vi "Simple TCP - Client_draft 1.vi"() -> ()   [LabVIEW 2021]
doc: "Demonstrates how to open a connection to an TCP server, read the data being sent, and display the data on a chart. This VI is designed to stop if the TCP connection is terminated."
uses:
  <vilib>/Analysis/3filter.llb/Butterworth Filter (DBL).vi
  <vilib>/Analysis/NI_AALBase.lvlib
  <vilib>/ptbypt/NI_PtbyPt.lvlib
panel:
  in  "Server Closed":string="The server VI closed the connection."
  in  "error in (no error)":errorcluster
  out "Waveform Graph":dbl[](graph)
  in  "Stop":bool
  in  "Boolean":bool
  out "Waveform Graph 2":dynamicdata(graph)
  out "Waveform Graph 3":dbl[](graph)
  out "Waveform Graph 4":dynamicdata(graph)
  out "Waveform Graph 5":dynamicdata(graph)
  out "Waveform Graph 6":dynamicdata(graph)
  out "Array Size":u32
  out "Waveform Graph 7":dynamicdata(graph)
  out "Waveform Graph 10":dynamicdata(graph)
  out "Array Size 3":u32
  # "Overview: Demonstrates the use of the TCP functions to connect to a TCP server VI and receive data.\nInstructions:\n1. Ensure Simple TCP - Server.vi is already running.\n2. Run the VI.\n3. Click Stop to stop the VI. Note that if you stop the server VI, this VI will stop automatically."
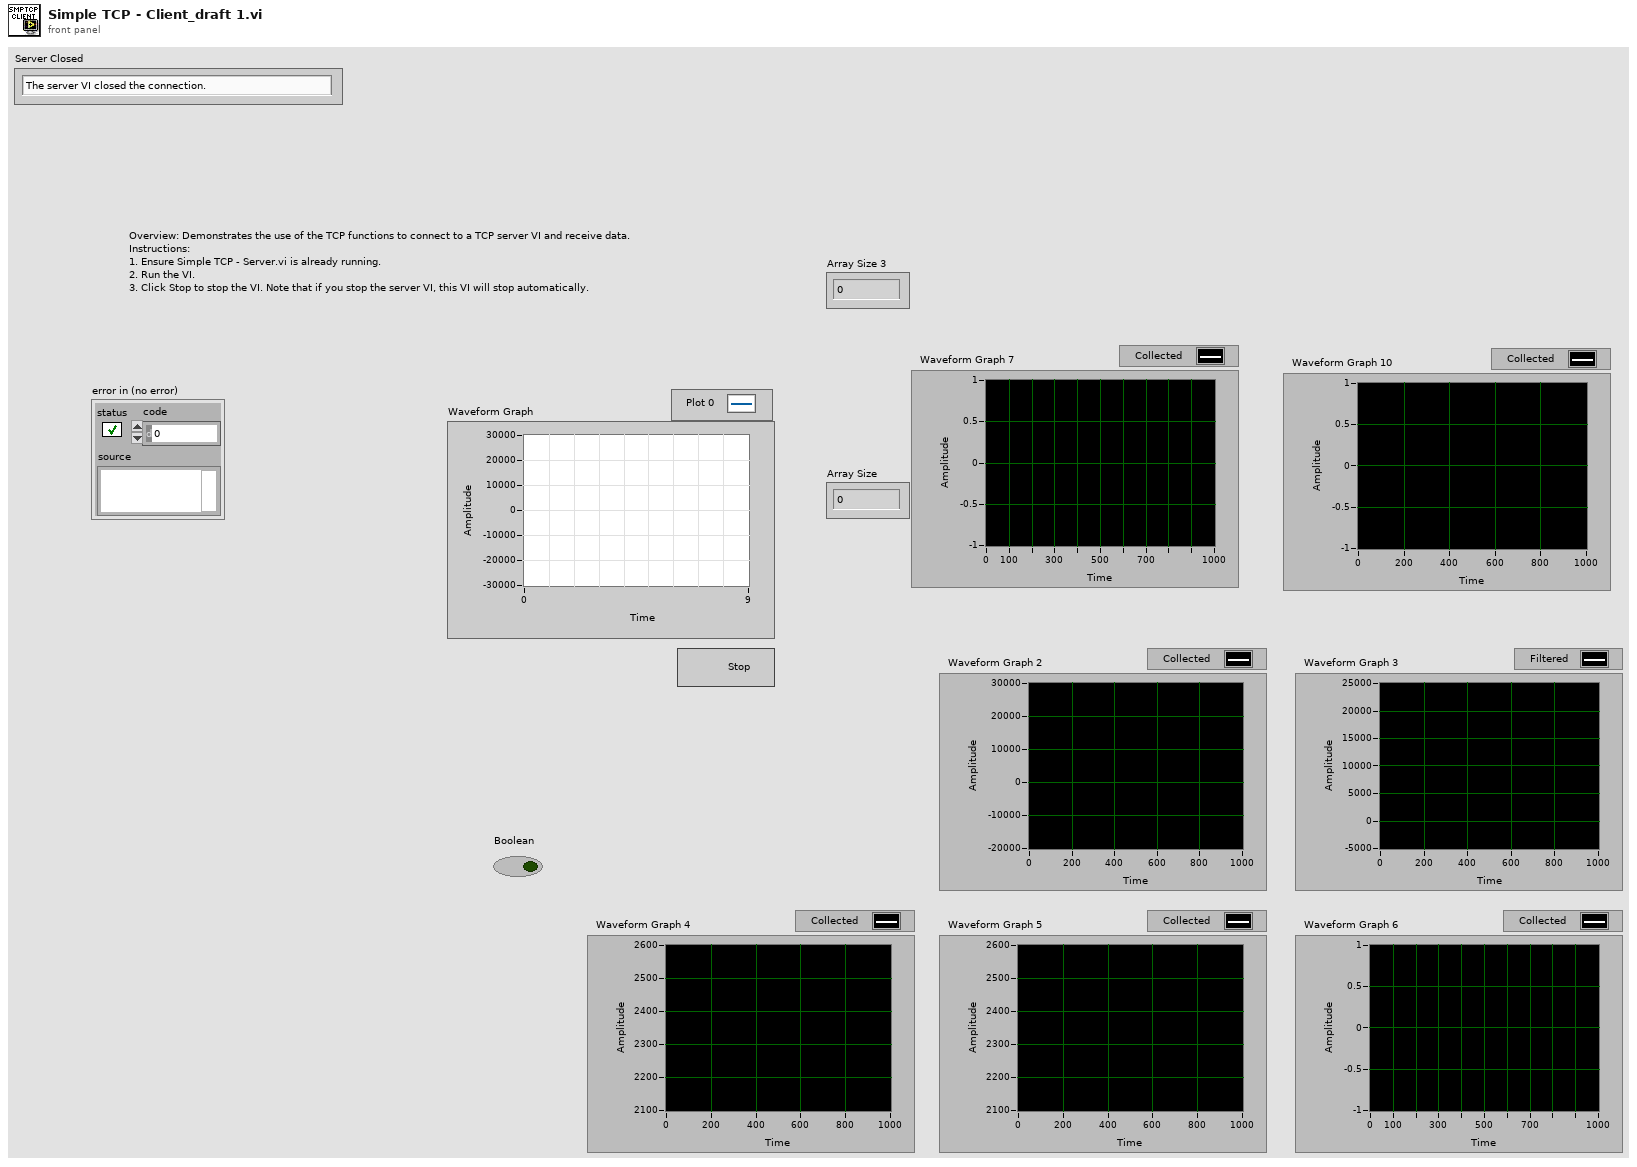
[diagram p1: front panel]
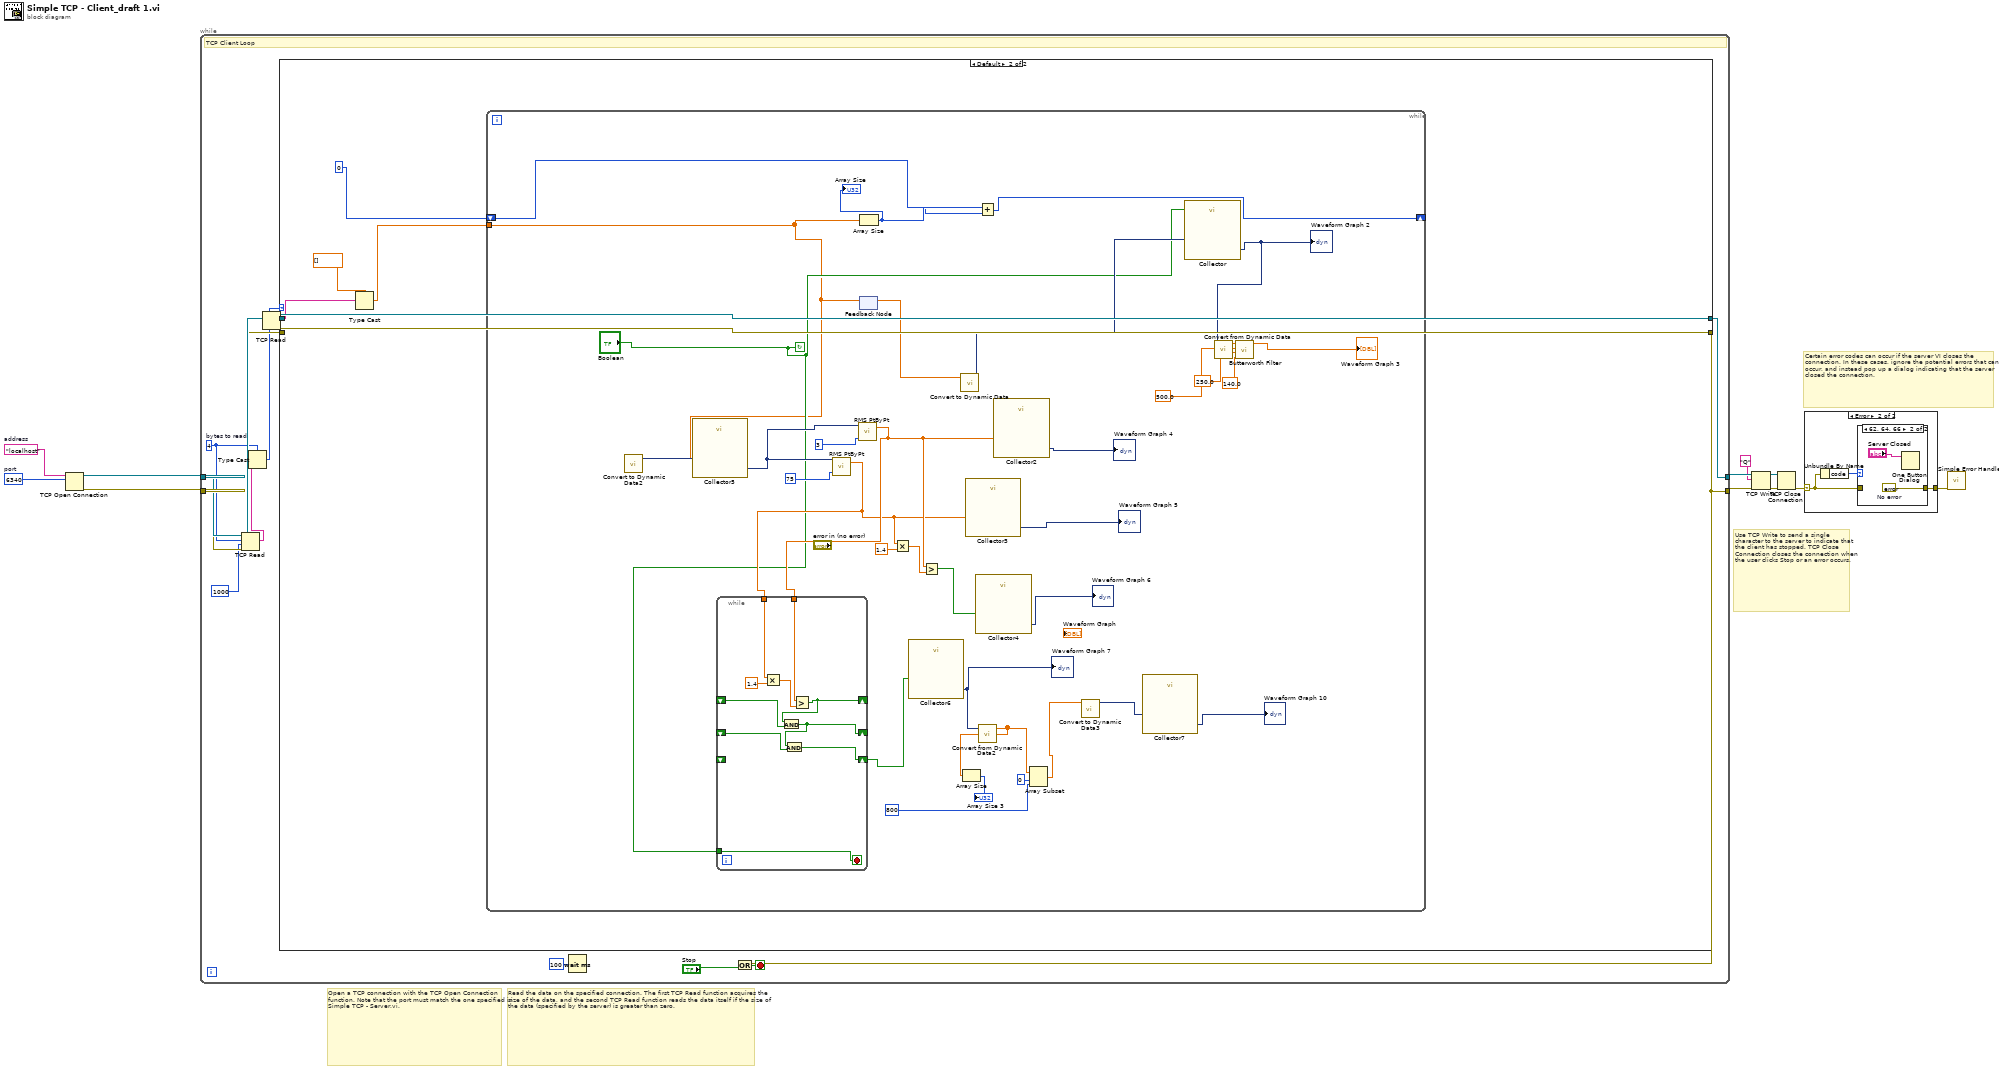
[diagram p0: block diagram]
diagram:
  w1 = u16 6340  # port
  w2 = "localhost"  # address
  # "Certain error codes can occur if the server VI closes the connection. In these cases, ignore the potential errors that can occur, and instead pop up a dialog indicating that the server closed the connection."
  # "Use TCP Write to send a single character to the server to indicate that the client has stopped. TCP Close Connection closes the connection when the user clicks Stop or an error occurs."
  # "Read the data on the specified connection. The first TCP Read function acquires the size of the data, and the second TCP Read function reads the data itself if the size of the data (specified by the server) is greater than zero."
  # "Open a TCP connection with the TCP Open Connection function. Note that the port must match the one specified in Simple TCP - Server.vi."
  n1 = TCP Open Connection(address=w2, remote port or service name=w1) -> (connection ID=w11:refnum<k5>, error out=w10:errorcluster)  [unwired: 3 in]
  n2 = while {
    tunnel: w10 -> [w20]
    tunnel: w11 -> [w21]
    tunnel: [w16] -> w8
    tunnel: [w15] -> w6
    stop <- w18 stop-if-true
    w19 = 4  # bytes to read
    # "TCP Client Loop"
    n3 = TCP Read(connection ID=w21, bytes to read=w19, error in (no error)=w20, 9:1000 ("timeout ms (25000)")) -> (connection ID out=w23:refnum<k5>, data out=w24:string, error out=w22:errorcluster)  [unwired: 1 in]
    n4 = Type Cast(type=w19, x=w24) -> (*(type *) &x=w14:i32)
    n5 = case shown="Default" w14 {
      selector: w14 -> [_ w29]
      tunnel: w23 -> [w26 w35]
      tunnel: w22 -> [w25 w34]
      tunnel: [w26 w32] -> w16
      tunnel: [w25 w31] -> w15
      frame ..0 {
        # "The server has not written any data"
      }
      frame Default {
        n6 = TCP Read(connection ID=w35, bytes to read=w29, error in (no error)=w34) -> (connection ID out=w32:refnum<k5>, data out=w30:string, error out=w31:errorcluster)  [unwired: 2 in]
        n7 = Type Cast(type=dbl[] [] ("chart"), x=w30) -> (*(type *) &x=w27:dbl[])
        n8 = while {
          shift-right: [w49] -> _
          shift-left: 0 -> [w50]
          tunnel: w27 -> [w36]
          stop <- "Boolean" continue-if-true
          n9 = call "Convert to Dynamic Data2"("Array"=w36) -> ("Dynamic Data Type"=w54:dynamicdata)  [unwired: 3 in]
          n10 = call "Collector5"("Signals"=w54) -> ("Collected Signals"=w53:dynamicdata)  [unwired: 9 in, 1 out]
          n11 = call <vilib>:"RMS PtByPt.vi"("sample length"=75, "x"=w53) -> ("rms value"=w47:dbl)  [unwired: 2 in, 1 out]
          n12 = call <vilib>:"RMS PtByPt.vi"("sample length"=3, "x"=w53) -> ("rms value"=w48:dbl)  [unwired: 2 in, 1 out]
          n13 = while {
            tunnel: w48 -> [w77]
            tunnel: w47 -> [w76]
            shift-right: [w71] -> _
            shift-left: _ -> [w72]
            shift-right: [w74] -> _
            shift-left: _ -> [w73]
            tunnel: "Boolean" -> [w75]
            shift-right: [w70] -> w44
            shift-left: _ -> [_]
            stop <- w75 stop-if-true
            n14 = Multiply(x=w76, y=1.4) -> (x*y=w78:dbl)
            n15 = Greater?(x=w77, y=w78) -> (0:w74:bool)
            n16 = And(x=w74, y=w73) -> (x .and. y?=w71:bool)
            n17 = And(x=w71, y=w72) -> (x .and. y?=w70:bool)
          }
          n18 = feedback-in #1(w36) -> ()
          n19 = feedback #1() -> (w52:dbl[])  [unwired: 1 in]
          n20 = Array Size(array=w36) -> (size(s)=w51:i32)
          "Array Size" <- w51
          n21 = Multiply(x=w47, y=1.4) -> (x*y=w57:dbl)
          n22 = call "Collector6"("Signals"=w44) -> ("Collected Signals"=w42:dynamicdata)  [unwired: 9 in, 1 out]
          "Waveform Graph 7" <- w42
          n23 = Greater?(x=w48, y=w57) -> (0:w56:bool)
          n24 = call "Convert to Dynamic Data"("Array"=w52) -> ("Dynamic Data Type"=w61:dynamicdata)  [unwired: 3 in]
          n25 = call "Collector3"("Signals"=w47) -> ("Collected Signals"=→"Waveform Graph 5":dynamicdata)  [unwired: 9 in, 1 out]
          n26 = call "Collector4"("Signals"=w56) -> ("Collected Signals"=→"Waveform Graph 6":dynamicdata)  [unwired: 9 in, 1 out]
          n27 = call "Convert from Dynamic Data2"("Dynamic Data Type"=w42) -> ("Array"=w39:dbl[])  [unwired: 3 in]
          n28 = Array Size(array=w39) -> (size(s)=→"Array Size 3":i32)
          n29 = Add(x=w51, y=w50) -> (x+y=w49:i32)
          n30 = call "Collector2"("Signals"=w48) -> ("Collected Signals"=→"Waveform Graph 4":dynamicdata)  [unwired: 9 in, 1 out]
          n31 = Array Subset(array=w39, index=0, length=800 ("index")) -> (w37:dbl[])
          n32 = call "Convert to Dynamic Data3"("Array"=w37) -> ("Dynamic Data Type"=w43:dynamicdata)  [unwired: 3 in]
          n33 = call "Collector7"("Signals"=w43) -> ("Collected Signals"=→"Waveform Graph 10":dynamicdata)  [unwired: 9 in, 1 out]
          n34 = call "Collector"("Enable"="Boolean", "Signals"=w61) -> ("Collected Signals"=w64:dynamicdata)  [unwired: 8 in, 1 out]
          "Waveform Graph 2" <- w64
          n35 = call "Convert from Dynamic Data"("Dynamic Data Type"=w64) -> ("Array"=w66:dbl[])  [unwired: 3 in]
          n36 = call-poly <vilib>:"Butterworth Filter.vi"("low cutoff freq: fl"=140.0, "high cutoff freq: fh"=250.0, "sampling freq: fs"=500.0, "X"=w66) -> ("Filtered X"=→"Waveform Graph 3":dbl[])  [unwired: 4 in, 1 out]
        }
      }
    }
    n37 = Wait (ms)(milliseconds to wait=u32 100) -> ()  [unwired: 1 out]
    n38 = Or(x=w15, y="Stop") -> (x .or. y?=w18:bool)
  }
  n39 = TCP Write(connection ID=w8, data in="Q", error in (no error)=w6) -> (connection ID out=w9:refnum<k5>, error out=w7:errorcluster)  [unwired: 2 out]
  n40 = TCP Close Connection(connection ID=w9, error in (no error)=w7) -> (error out=w4:errorcluster)  [unwired: 1 in, 1 out]
  n41 = case shown="Error" w4 {
    selector: w4 -> [w80 w82]
    tunnel: [w80 w81] -> w3
    frame No Error {
    }
    frame Error {
      n42 = Unbundle By Name(w82) -> ("code"=w83:i32)
      n43 = case shown="62, 64, 66" w83 {
        tunnel: w82 -> [w84 _]
        tunnel: [w84 w86] -> w81
        frame Default {
        }
        frame 62, 64, 66 {
          w86 = errorcluster {"status"=FALSE, "code"=0, "source"=""}  # No error
          n44 = One Button Dialog(message="Server Closed") -> ()  [unwired: 1 in, 1 out]
        }
      }
    }
  }
  n45 = call <vilib>:"Simple Error Handler.vi"("error in (no error)"=w3) -> ()  [unwired: 4 in, 5 out]
